vi "DLLTryFiles.vi"() -> ()   [LabVIEW 2020]
uses:
  <vilib>/Utility/file.llb/Read Delimited Spreadsheet (DBL).vi
panel:
  in  "Путь до .exe файла":path
  in  "Текущее действие":T1(ring)
  out "Intensity Graph":dbl[][](graph)
  in  "Путь до выходного файла":path
  in  "Сюда сохранится система":path
  in  "System":string
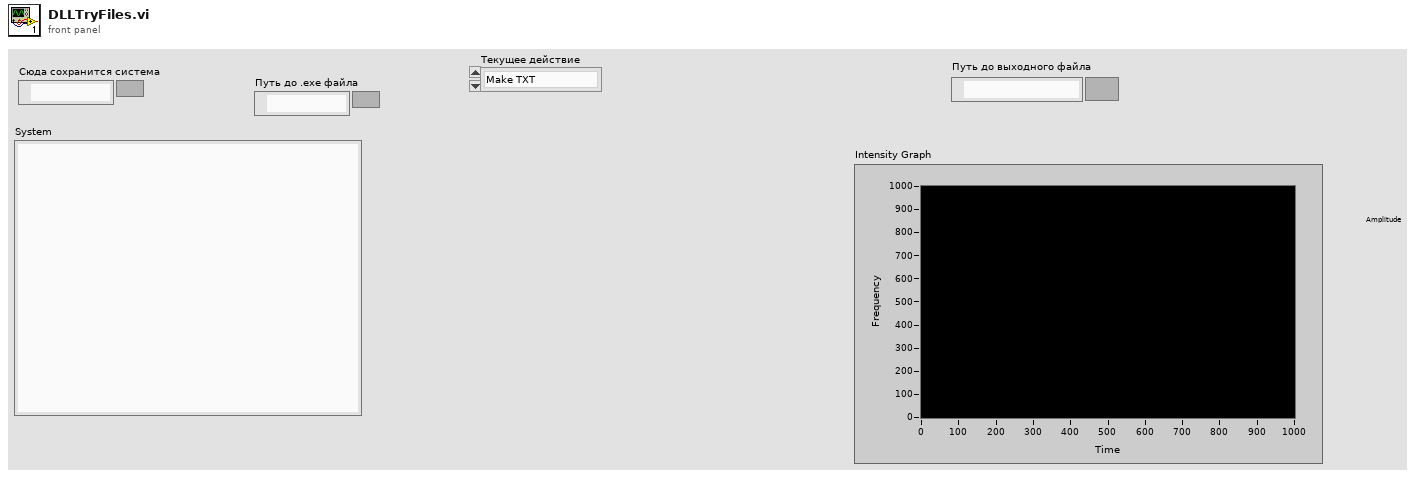
[diagram p1: front panel]
types:
  T1 = enum16{"Make TXT", "Run shell", "Run analysis", "Read csv"}
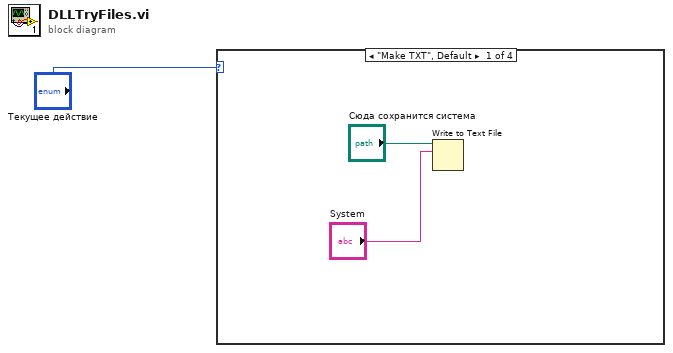
[diagram p0: block diagram]
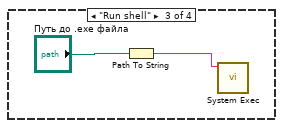
[diagram p3: hidden frame]
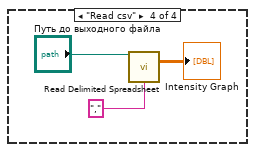
[diagram p4: hidden frame]
diagram:
  n1 = case shown="\"Make TXT\", Default" "Текущее действие" {
    frame "Make TXT", Default {
      n2 = Write to Text File(file (use dialog)="Сюда сохранится система", text="System") -> ()  [unwired: 2 in, 3 out]
    }
    frame "Run analysis" {
    }
    frame "Run shell" {
      n3 = Path To String(path="Путь до .exe файла") -> (string=w4:string)
      n4 = call <vilib>:"System Exec.vi"("command line"=w4) -> ()  [unwired: 7 in, 4 out]
    }
    frame "Read csv" {
      n5 = call-poly <vilib>:"Read Delimited Spreadsheet.vi"("file path (dialog if empty)"="Путь до выходного файла", "delimiter (\\t)"="," ("delimiter (\\t)")) -> ("all rows"=→"Intensity Graph":dbl[][])  [unwired: 8 in, 5 out]
    }
  }
